vi "XIPIN_RGB_to_YCrCb_Color-Space_Converter_4_0.vi"   [LabVIEW 2017]
doc: "The Xilinx RGB to YCrCb Color Space Converter LogiCORE with built-in support for 5 formats and 3 range standards. The implementation is a simplified 3x3 constant coefficient matrix multiplier, which uses only 4 multipliers exploiting the inter-relations of RGB to YCrCb coefficients. The module is optimized to take advantage of multiply-add capabilities of DSP slices.\n------------------------------------\n<b>Need License</b> : No"
uses:
  <vilib>/rvi/XilinxIP/XIPIN_XNode/niFpgaXIPIN.xnode
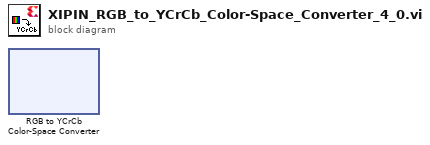
[diagram p0: block diagram]
diagram:
  n1 = xnode ("RGB to YCrCb Color-Space Converter")() -> ()
